vi "GetViCtrlRefGen.vi"(8 "ErrorIn(No Error)":errorcluster caption="entrée d'erreur (pas d'erreur)", 10 "InclTabCTrl":bool, 11 "VIRef":refnum<vi>) -> (0 "sortie d'erreur":errorcluster, 2 "ControlsRefs":refnum<vi>[](array[refnum]), 3 "ControlsNames":string[](array[string]))   [LabVIEW 2019]
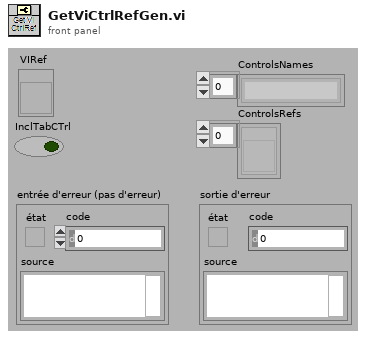
[diagram p1: front panel]
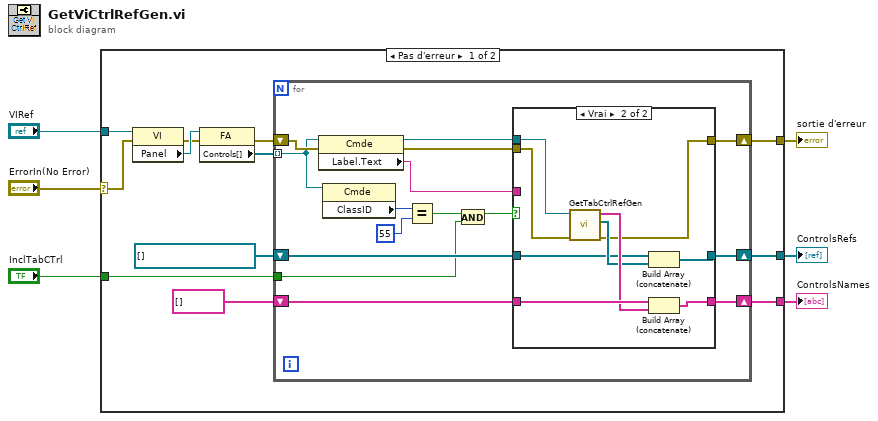
[diagram p0: block diagram]
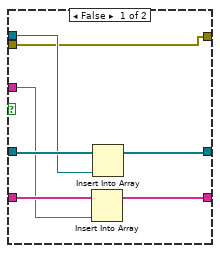
[diagram p2: hidden frame]
diagram:
  n1 = case shown="Pas d'erreur" "ErrorIn(No Error)" {
    selector: "ErrorIn(No Error)" -> [w14 w50]
    tunnel: [w10 w50] -> w5
    tunnel: "VIRef" -> [w16 _]
    tunnel: [w12 _] -> w3
    tunnel: [w11 _] -> w2
    tunnel: "InclTabCTrl" -> [w9 _]
    frame No Error {
      n2 = property class="VI"(reference=w16, error in=w14) -> (error out=w17:errorcluster, "Panel"=w18:refnum<vi>)  [unwired: 1 out]
      n3 = property class="FA"(reference=w18, error in=w17) -> (error out=w13:errorcluster, "Controls[]"=w15:refnum<vi>[])  [unwired: 1 out]
      n4 = for {
        tunnel: w15 -> [w32] mode=indexing
        shift-right: [w21] -> w10
        shift-left: w13 -> [w33]
        shift-right: [w26] -> w12
        shift-left: refnum<vi>[] [] -> [w25]
        shift-right: [w24] -> w11
        shift-left: string[] [] -> [w22]
        tunnel: w9 -> [w19]
        n5 = property class="Cmde"(reference=w32, error in=w33) -> (reference out=w28:refnum<vi>, error out=w23:errorcluster, "Label.Text"=w29:string)
        n6 = property class="Cmde"(reference=w32) -> ("ClassID"=w31:u32)  [unwired: 1 in, 2 out]
        n7 = Equal?(x=w31, y=u32 55) -> (x = y?=w27:bool)
        n8 = And(x=w27, y=w19) -> (x .and. y?=w20:bool)
        n9 = case shown="Vrai" w20 {
          tunnel: w29 -> [w36 _]
          tunnel: w28 -> [w35 w49]
          tunnel: [w40 w45] -> w26
          tunnel: w25 -> [w39 w43]
          tunnel: [w38 w46] -> w24
          tunnel: w23 -> [w34 w42]
          tunnel: w22 -> [w37 w48]
          tunnel: [w34 w41] -> w21
          frame False {
            n10 = Insert Into Array(array=w37, new element=w36) -> (w38:string[])  [unwired: 1 in]
            n11 = Insert Into Array(array=w39, new element=w35) -> (w40:refnum<vi>[])  [unwired: 1 in]
          }
          frame True {
            n12 = call <userlib>:"GetTabCtrlRefGen.vi"("ErrorIn(No Error)"=w42, "CommandRef"=w49) -> ("sortie d'erreur"=w41:errorcluster, "ControlsRefs"=w44:refnum<vi>[], "ControlsNames"=w47:string[])  [unwired: 7 in]
            n13 = Build Array (concatenate)(w43, w44) -> (w45:refnum<vi>[])
            n14 = Build Array (concatenate)(w48, w47) -> (w46:string[])
          }
        }
      }
    }
    frame Error {
    }
  }
  "sortie d'erreur" <- w5
  "ControlsNames" <- w2
  "ControlsRefs" <- w3
